vi "Pre Launch Init.vi"(11 "Nested in":refnum<class "MSS Host Actor.lvclass">) -> (0 "error out":errorcluster, 3 "Nested out":refnum<class "MSS Host Actor.lvclass">)   [LabVIEW 2023, in "MSS Host Actor.lvlib" / "MSS Host Actor.lvclass"]
doc: "(<B>Filename</B>: Actor Framework.lvlib:Actor.lvclass:Pre Launch Init.vi)\n\nDefines behavior that occurs after the Launch Nested Actor method is invoked but before the actor's Actor Core method begins running.\n\nBy default, this method does nothing. A descendant class may override it to define behavior."
uses:
  MSS Host Actor.lvclass
  C:/Program Files/National Instruments/LabVIEW 2023/vi.lib/ActorFramework/Actor/Actor.lvclass
  MSS Host Actor.lvclass/MSS Host Actor.ctl
  <vilib>/ActorFramework/Actor/Actor.lvclass
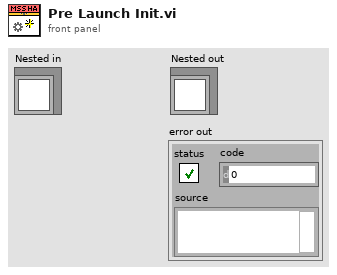
[diagram p1: front panel]
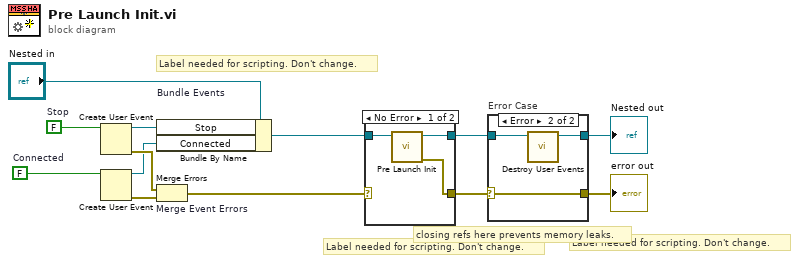
[diagram p0: block diagram]
diagram:
  w4 = FALSE  # Connected
  w13 = FALSE  # Stop
  # "Label needed for scripting. Don't change."
  # "Label needed for scripting. Don't change."
  # "Label needed for scripting. Don't change."
  # "closing refs here prevents memory leaks."
  n1 = Create User Event(user event datatype=w13) -> (user event=w10:refnum<user-event>, error out=w12:errorcluster)  [unwired: 1 in]
  n2 = Create User Event(user event datatype=w4) -> (user event=w3:refnum<user-event>, error out=w2:errorcluster)  [unwired: 1 in]
  n3 = Bundle By Name "Bundle Events"(cluster="Nested in", "Stop"=w10, "Connected"=w3) -> (w7:refnum<class "MSS Host Actor.lvclass">)
  n4 = Merge Errors "Merge Event Errors"(w12, w2) -> (w6:errorcluster)
  n5 = case shown="No Error" w6 {
    selector: w6 -> [_ w18]
    tunnel: [w16 w17] -> w8
    tunnel: w7 -> [w15 w17]
    tunnel: [w14 w18] -> w5
    frame No Error {
      n6 = call-parent "Pre Launch Init.vi"("Actor in"=w15) -> ("error out"=w14:errorcluster, "Actor out"=w16:refnum<class "MSS Host Actor.lvclass">)  [unwired: 9 in]
    }
    frame Error {
    }
  }
  n7 = case "Error Case" shown="Error" w5 {
    selector: w5 -> [w19 w23]
    tunnel: w8 -> [w20 w22]
    tunnel: [w20 w21] -> w11
    tunnel: [w19 w23] -> w9
    frame No Error {
    }
    frame Error {
      n8 = call "Destroy User Events.vi"("UI Template in"=w22) -> ("UI Template out"=w21:refnum<class "MSS Host Actor.lvclass">)  [unwired: 10 in]
    }
  }
  "error out" <- w9
  "Nested out" <- w11
